vi "Read ListBox Selected Tests and Order.vi"(8 "Error In":errorcluster, 11 "Experiment Cluster":refnum<vi>) -> (0 "Error Out":errorcluster, 1 "Per Exp Tests to Run":string[](array[string]), 2 "Meas_Type for Display":T1=[0, 2, 4], 3 "Item Names for Display":string[](array[string]))   [LabVIEW 2013]
uses:
  Controls/Individual User Inputs_MultiTest.ctl
  Controls/Test Selection.ctl
panel:
  # "Calculation Settings"
  # "Test Settings"
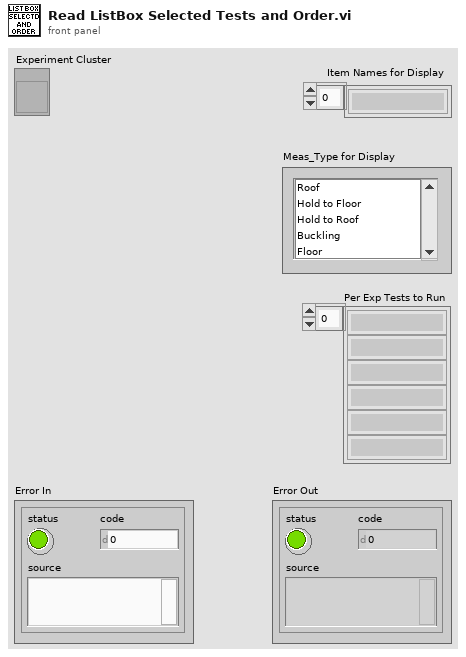
[diagram p1: front panel]
types:
  T1 = typedef "Test Selection.ctl" = i32[]
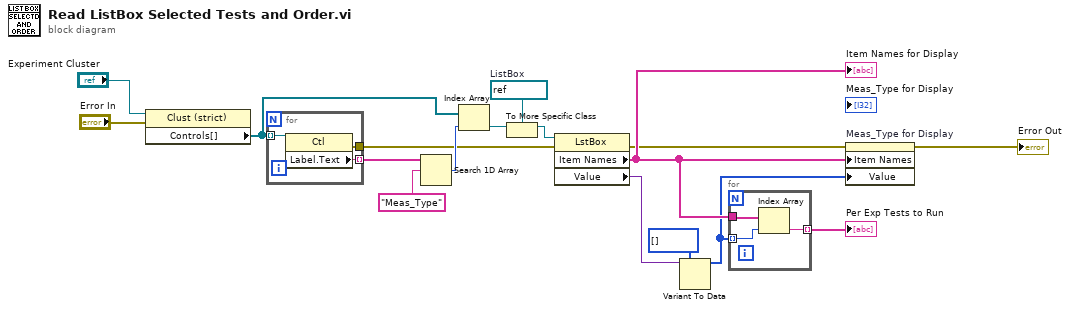
[diagram p0: block diagram]
diagram:
  w16 = refnum<vi> refnum  # ListBox
  n1 = property class="Clust (strict)"(reference="Experiment Cluster", error in="Error In") -> ("Controls[]"=w14:refnum<vi>[])  [unwired: 2 out]
  n2 = for {
    tunnel: w14 -> [w20] mode=indexing
    tunnel: [w19] -> w11
    tunnel: [w18] -> w10 mode=indexing
    n3 = property class="Ctl"(reference=w20) -> (error out=w19:errorcluster, "Label.Text"=w18:string)  [unwired: 1 in, 1 out]
  }
  n4 = Search 1D Array(1D array=w10, element="Meas_Type") -> (index of element=w13:i32)  [unwired: 1 in]
  n5 = Index Array(array=w14, index=w13) -> (element=w15:refnum<vi>)
  n6 = To More Specific Class(target class=w16, reference=w15) -> (specific class reference=w17:refnum<vi>)  [unwired: 1 in, 1 out]
  n7 = property class="LstBox"(reference=w17, error in=w11) -> (error out=w4:errorcluster, "Item Names"=w6:string[], "Value"=w9:variant)  [unwired: 1 out]
  "Item Names for Display" <- w6
  n8 = Variant To Data(type=i32[] [] ("Meas_Type"), Variant=w9) -> (data=w5:i32[])  [unwired: 1 in, 1 out]
  n9 = for {
    tunnel: w5 -> [w22] mode=indexing
    tunnel: w6 -> [w23]
    tunnel: [w21] -> w7 mode=indexing
    n10 = Index Array(array=w23, index=w22) -> (element=w21:string)
  }
  "Per Exp Tests to Run" <- w7
  n11 = property on="Meas_Type for Display" class="LstBox (strict)"(error in=w4, "Item Names"=w6, "Value"=w5) -> (error out=→"Error Out":errorcluster)  [unwired: 1 in, 1 out]
